vi "UI.vi"() -> ()   [LabVIEW 2020]
uses:
  <vilib>/addons/_JKI.lib/REST Client/classes/REST Client/HTTP Header.ctl
  Globals.vi
  <vilib>/addons/_JKI.lib/REST Client/classes/REST Client/REST Client.lvclass
panel:
  out "Response":string
  in  "Button":bool
  in  "Prompt":string
  # "Your Prompt Here"
  # "ChatGPT Response"
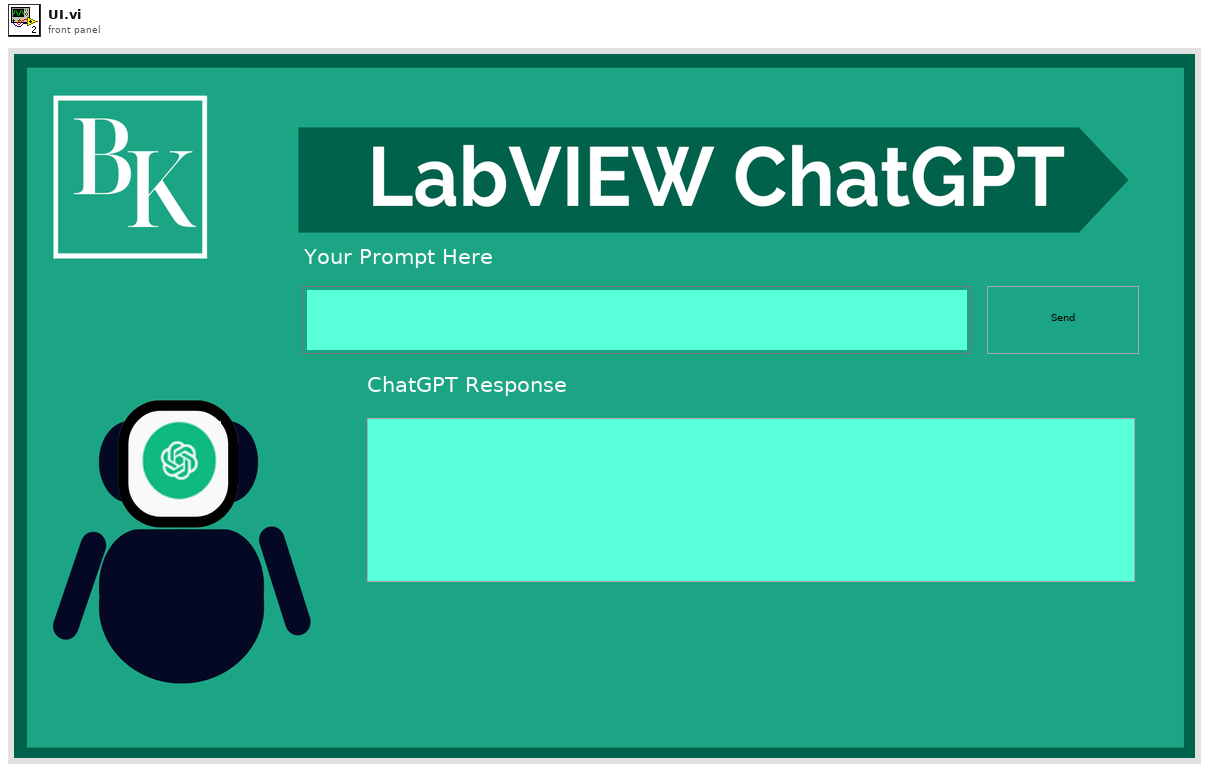
[diagram p1: front panel]
types:
  T1 = typedef "REST Client.lvlib/REST Client.lvclass/HTTP Header.ctl" = cluster{"header":string, "value":string}
  T2 = cluster{"id":string, "object":string, "created":i32, "model":string, "choices":cluster{"index":i32, "message":cluster{"role":string, "content":string}, "finish_reason":string}[], "usage":cluster{"prompt_tokens":i32, "completion_tokens":i32, "total_tokens":i32}}
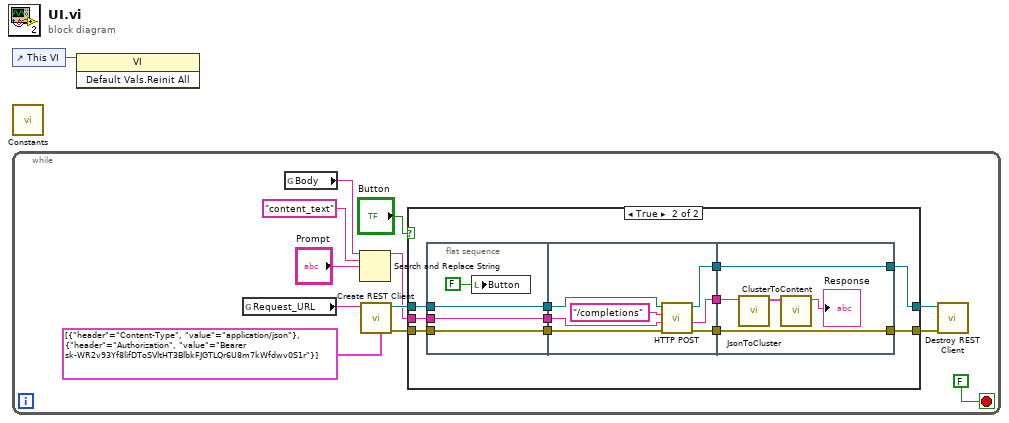
[diagram p0: block diagram]
diagram:
  n1 = control-ref of="This VI"() -> (w1:refnum<vi>)
  n2 = call "Constants.vi"() -> ()  [unwired: 12 in]
  n3 = while {
    stop <- FALSE stop-if-true
    n4 = global read "Globals.vi" "Request_URL"() -> (w5:string)
    n5 = global read "Globals.vi" "Body"() -> (w4:string)
    n6 = Search and Replace String(input string=w4, search string="content_text" ("substring (\"\")"), replace string="Prompt") -> (result string=w9:string)  [unwired: 5 in, 3 out]
    n7 = call <vilib>:"Create REST Client.vi"("Default Headers ([JSON])"=T1[] [{"header"="Content-Type", "value"="application/json"}, {"header"="Authorization", "value"="Bearer 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"}], "Base URL"=w5) -> ("error out"=w13:errorcluster, "REST Client out"=w12:refnum<class "REST Client.lvclass">)  [unwired: 8 in]
    n8 = case shown="True" "Button" {
      tunnel: w13 -> [w15 w26]
      tunnel: w12 -> [w14 w25]
      tunnel: w9 -> [_ w24]
      tunnel: [w15 w20] -> w3
      tunnel: [w14 w17] -> w2
      frame False {
      }
      frame True {
        n9 = flat-sequence {
          tunnel: w24 -> [w28]
          tunnel: w25 -> [w29]
          tunnel: w26 -> [w30]
          tunnel: [w30] -> w23
          tunnel: [w29] -> w22
          tunnel: [w28] -> w21
          tunnel: w23 -> [w34]
          tunnel: w22 -> [w36]
          tunnel: w21 -> [w35]
          tunnel: [w33] -> w19
          tunnel: [w32] -> w18
          tunnel: [w31] -> w16
          tunnel: [w40] -> w20
          tunnel: w19 -> [w40]
          tunnel: w18 -> [w39]
          tunnel: [w38] -> w17
          tunnel: w16 -> [w38]
          frame #0 {
            n10 = local write "Button"(FALSE ("Button")) -> ()
          }
          frame #1 {
            n11 = call-dynamic "HTTP POST.vi"("error in (no error)"=w34, "Request body"=w35, "Path"="/completions", "REST Client in"=w36) -> ("error out"=w33:errorcluster, "Response body"=w32:string, "REST Client out"=w31:refnum<class "REST Client.lvclass">)  [unwired: 2 in, 3 out]
          }
          frame #2 {
            n12 = call "JsonToCluster.vi"("Response body"=w39) -> ("Cluster"=w42:T2)  [unwired: 10 in]
            n13 = call "ClusterToContent.vi"("Cluster"=w42) -> ("Content"=→"Response":string)  [unwired: 10 in]
          }
        }
      }
    }
    n14 = call-dynamic "Destroy REST Client.vi"("error in (no error)"=w3, "REST Client in"=w2) -> ()  [unwired: 9 in, 1 out]
  }
  n15 = invoke class="VI" method="Default Vals.Reinit All"(reference=w1) -> ()  [unwired: 2 in, 3 out]
